vi "alert.vi"(2 "error in":errorcluster, 3 "Path":path=path "alert_sound.wav", 4 "Turn on":bool) -> (0 "error out":errorcluster)   [LabVIEW 2017]
panel:
  in  "device ID":u32 format="%.0x"
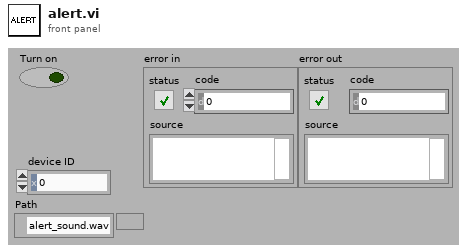
[diagram p1: front panel]
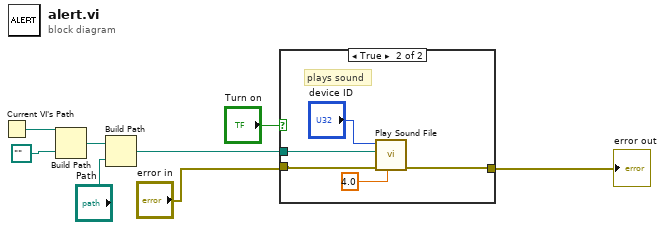
[diagram p0: block diagram]
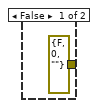
[diagram p2: hidden frame]
diagram:
  n1 = Current VI's Path() -> (path=w6:path)
  n2 = Build Path(base path=w6, name or relative path=path "..") -> (appended path=w4:path)
  n3 = Build Path(base path=w4, name or relative path="Path") -> (appended path=w2:path)
  n4 = case shown="True" "Turn on" {
    tunnel: w2 -> [_ w14]
    tunnel: "error in" -> [_ w13]
    tunnel: [errorcluster {"status"=FALSE, "code"=0, "source"=""} ("error out") w12] -> w7
    frame False {
    }
    frame True {
      # "plays sound"
      n5 = call <vilib>:"Play Sound File.vi"("timeout (sec)"=4.0, "error in (no error)"=w13, "path"=w14, "device ID"="device ID") -> ("error out"=w12:errorcluster)  [unwired: 6 in, 1 out]
    }
  }
  "error out" <- w7
